vi "ABS_Move(PAB).vi"(5 "baud rate (9600)":u32=115200 caption="보 전송속도(9600)", 6 "Y Position(ABS)":dbl format="%#_8g", 7 "X Position(ABS)":dbl format="%#_8g", 8 "Port":refnum<visa-resource-name>="COM4" caption="VISA 리소스 이름") -> (2 "에러 출력":errorcluster, 3 "VISA 리소스 이름 출력":refnum<visa-resource-name>, 4 "연결된 문자열":string)   [LabVIEW 2016]
uses:
  <vilib>/Instr/_visa.llb/VISA Configure Serial Port (Instr).vi
  <vilib>/Instr/_visa.llb/VISA Flush IO Buffer Mask.ctl
panel:
  out "Write data":u32
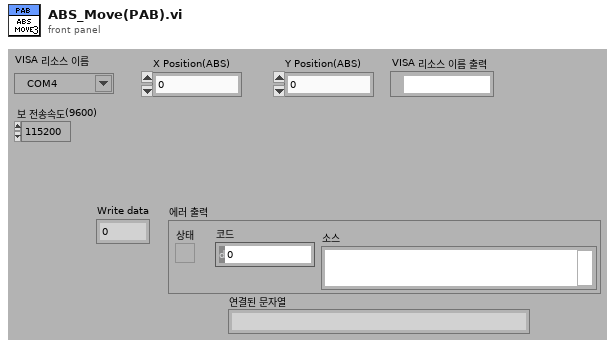
[diagram p1: front panel]
types:
  T1 = typedef "VISA Flush IO Buffer Mask.ctl" = u16
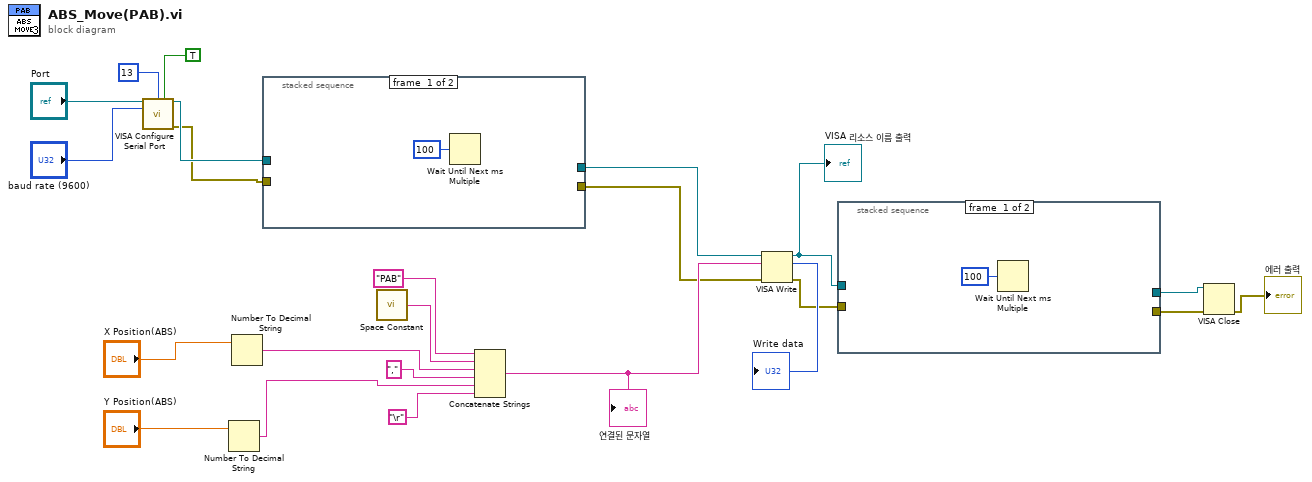
[diagram p0: block diagram]
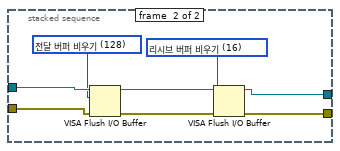
[diagram p2: hidden frame]
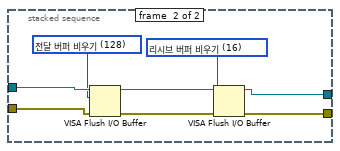
[diagram p3: hidden frame]
diagram:
  n1 = call-poly "VISA Configure Serial Port"("VISA resource name"="Port", "termination char\n(0xA = '\\n' = LF)"=i16 13 ("termination char\n(0xA = '\\n' = LF)"), "Enable Termination\nChar (T)"=TRUE ("Enable Termination\nChar (T)"), "baud rate (9600)"="baud rate (9600)") -> ("VISA resource name out"=w8:refnum<visa-resource-name>, "error out"=w7:errorcluster)  [unwired: 10 in]
  n2 = Number To Decimal String(number="Y Position(ABS)") -> (decimal integer string=w15:string)  [unwired: 1 in]
  n3 = Number To Decimal String(number="X Position(ABS)") -> (decimal integer string=w17:string)  [unwired: 1 in]
  n4 = stacked-sequence {
    tunnel: w8 -> [_ w32]
    tunnel: w7 -> [_ w31]
    tunnel: [_ w27] -> w6
    tunnel: [_ w26] -> w5
    frame #0 {
      n5 = Wait Until Next ms Multiple(millisecond multiple=u32 100 ("ms 배수")) -> ()  [unwired: 1 out]
    }
    frame #1 {
      w25 = T1 16 items=["리시브 버퍼 비우기"=16, "전달 버퍼 디바이스에 쓰기"=32, "리시브 버퍼 비우기(I/O 없음)"=64, "전달 버퍼 비우기"=128] ("Mask")
      w30 = T1 128 items=["리시브 버퍼 비우기"=16, "전달 버퍼 디바이스에 쓰기"=32, "리시브 버퍼 비우기(I/O 없음)"=64, "전달 버퍼 비우기"=128] ("Mask")
      n6 = VISA Flush I/O Buffer(VISA resource name=w32, mask (16)=w30, error in (no error)=w31) -> (VISA resource name out=w29:refnum<visa-resource-name>, error out=w28:errorcluster)
      n7 = VISA Flush I/O Buffer(VISA resource name=w29, mask (16)=w25, error in (no error)=w28) -> (VISA resource name out=w27:refnum<visa-resource-name>, error out=w26:errorcluster)
    }
  }
  n8 = call <vilib>:"Space Constant.vi"() -> ("String"=w18:string)
  n9 = Concatenate Strings("PAB" ("버퍼 쓰기"), w18, w17, "," ("문자열"), w15, "\r") -> (w21:string)
  "연결된 문자열" <- w21
  n10 = VISA Write(VISA resource name=w6, write buffer=w21, error in (no error)=w5) -> (VISA resource name out=w4:refnum<visa-resource-name>, return count=→"Write data":u32, error out=w3:errorcluster)
  "VISA 리소스 이름 출력" <- w4
  n11 = stacked-sequence {
    tunnel: w4 -> [_ w41]
    tunnel: w3 -> [_ w40]
    tunnel: [_ w36] -> w2
    tunnel: [_ w35] -> w1
    frame #0 {
      n12 = Wait Until Next ms Multiple(millisecond multiple=u32 100 ("ms 배수")) -> ()  [unwired: 1 out]
    }
    frame #1 {
      w34 = T1 16 items=["리시브 버퍼 비우기"=16, "전달 버퍼 디바이스에 쓰기"=32, "리시브 버퍼 비우기(I/O 없음)"=64, "전달 버퍼 비우기"=128] ("Mask")
      w39 = T1 128 items=["리시브 버퍼 비우기"=16, "전달 버퍼 디바이스에 쓰기"=32, "리시브 버퍼 비우기(I/O 없음)"=64, "전달 버퍼 비우기"=128] ("Mask")
      n13 = VISA Flush I/O Buffer(VISA resource name=w41, mask (16)=w39, error in (no error)=w40) -> (VISA resource name out=w38:refnum<visa-resource-name>, error out=w37:errorcluster)
      n14 = VISA Flush I/O Buffer(VISA resource name=w38, mask (16)=w34, error in (no error)=w37) -> (VISA resource name out=w36:refnum<visa-resource-name>, error out=w35:errorcluster)
    }
  }
  n15 = VISA Close(VISA resource name=w2, error in (no error)=w1) -> (error out=→"에러 출력":errorcluster)
